vi "BuildTemplatePadLists.vi"() -> (1 "RealTime":string[](array[string]), 2 "Templates":string[](array[string]), 3 "ScratchPads":string[](array[string]), 5 "All Templates":string[](array[string]))   [LabVIEW 2022 SP3]
uses:
  Mic/Mic_Global.vi
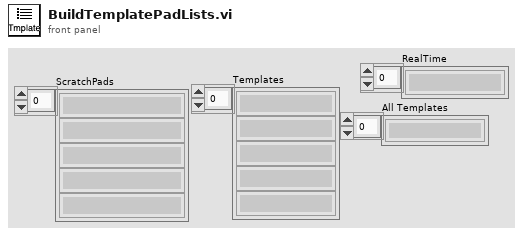
[diagram p1: front panel]
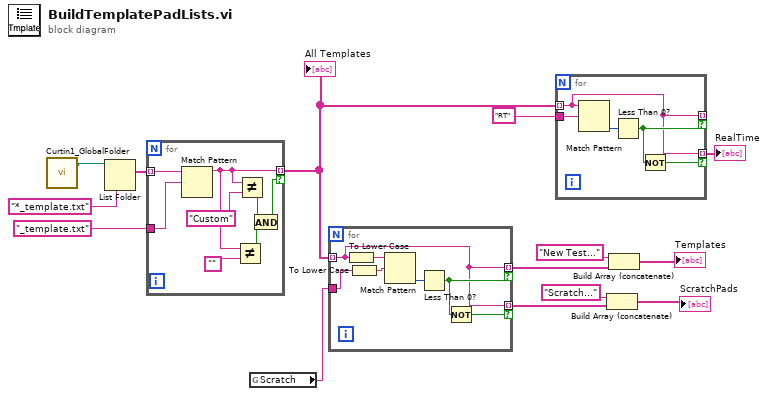
[diagram p0: block diagram]
diagram:
  n1 = call "Curtin1_GlobalFolder.vi"() -> ("LabVIEW Data Path"=w2:path)  [unwired: 1 in, 1 out]
  n2 = List Folder(path=w2, pattern="*_template.txt") -> (filenames=w3:string[])  [unwired: 2 in, 3 out]
  n3 = for {
    tunnel: w3 -> [w22] mode=indexing
    tunnel: [w19] -> w1 mode=indexing if=w15
    tunnel: "_template.txt" ("pattern") -> [w21]
    n4 = Match Pattern(string=w22, regular expression=w21) -> (before substring=w19:string)  [unwired: 4 out]
    n5 = Not Equal?(x=w19, y="") -> (x != y?=w17:bool)
    n6 = Not Equal?(x=w19, y="Custom") -> (x != y?=w16:bool)
    n7 = And(x=w16, y=w17) -> (x .and. y?=w15:bool)
  }
  "All Templates" <- w1
  n8 = global read "Mic_Global.vi" "Scratch"() -> (w13:string)
  n9 = for {
    tunnel: w1 -> [w25] mode=indexing
    tunnel: w13 -> [w29]
    tunnel: [w25] -> w7 mode=indexing if=w27
    tunnel: [w25] -> w11 mode=indexing if=w26
    n10 = To Lower Case(string=w25) -> (all lower case string=w24:string)
    n11 = To Lower Case(string=w29) -> (all lower case string=w23:string)
    n12 = Match Pattern(string=w24, regular expression=w23) -> (offset past match=w28:i32)  [unwired: 4 out]
    n13 = Less Than 0?(x=w28) -> (x < 0?=w27:bool)
    n14 = Not(x=w27) -> (.not. x?=w26:bool)
  }
  n15 = for {
    tunnel: w1 -> [w30] mode=indexing
    tunnel: "RT" ("regular expression") -> [w34]
    tunnel: [w30] -> _ mode=indexing if=w32
    tunnel: [w30] -> w12 mode=indexing if=w31
    n16 = Match Pattern(string=w30, regular expression=w34) -> (offset past match=w33:i32)  [unwired: 4 out]
    n17 = Less Than 0?(x=w33) -> (x < 0?=w32:bool)
    n18 = Not(x=w32) -> (.not. x?=w31:bool)
  }
  "RealTime" <- w12
  n19 = Build Array (concatenate)("Scratch..." ("y"), w11) -> (→"ScratchPads":string[])
  n20 = Build Array (concatenate)("New Test..." ("y"), w7) -> (→"Templates":string[])
